vi "Pre Launch Init.vi"(11 "Network Endpoint in":refnum<class "Network Endpoint.lvclass">) -> (0 "error out":errorcluster, 3 "Network Endpoint out":refnum<class "Network Endpoint.lvclass">)   [LabVIEW 2020, in "Network Endpoint.lvlib" / "Network Endpoint.lvclass"]
doc: "(<B>Filename</B>: Actor Framework.lvlib:Actor.lvclass:Pre Launch Init.vi)\n\nDefines behavior that occurs after the Launch Nested Actor method is invoked but before the actor's Actor Core method begins running.\n\nBy default, this method does nothing. A descendant class may override it to define behavior."
uses:
  Network Endpoint.lvclass
  Network Endpoint.lvclass/Network Endpoint.ctl
  Cache Manager/Cache Manager.lvclass/Cache Manager.ctl
  Serializer/Serializable Message/Serializable Msg.lvclass
  Cache Manager/Cache Manager.lvclass
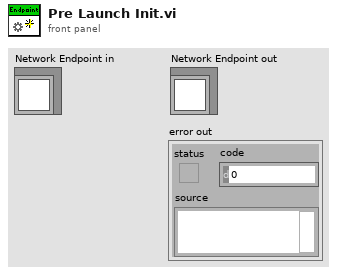
[diagram p1: front panel]
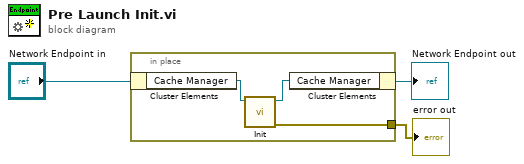
[diagram p0: block diagram]
diagram:
  n1 = in-place "In Place Element Structure" {
    in-place-border: [w4] -> w1
    n2 = in-place-cluster #1("Network Endpoint in") -> ("Cache Manager"=w6:refnum<class "Cache Manager.lvclass">)
    n3 = call "Init.vi"("Cache Manager DVR in"=w6) -> ("error out"=w4:errorcluster, "Cache Manager DVR out"=w5:refnum<class "Cache Manager.lvclass">)  [unwired: 9 in]
    n4 = in-place-cluster #1("Cache Manager"=w5) -> (→"Network Endpoint out":refnum<class "Network Endpoint.lvclass">)
  }
  "error out" <- w1
